vi "Test Method Result String when no Description Provided.vi"(8 "error in (no error)":errorcluster, 11 "Pass Assertion Test In":refnum<class "Method Result Test.lvclass">) -> (0 "error out":errorcluster, 3 "Pass Assertion Test Out":refnum<class "Method Result Test.lvclass">)   [LabVIEW 2020, in "LUnit Tests.lvlib" / "Method Result Test.lvclass"]
uses:
  Method Result Test.lvclass
  66165e44-9c0b-45c8-83e1-30937f51105d.vi
panel:
  out "Result String":string
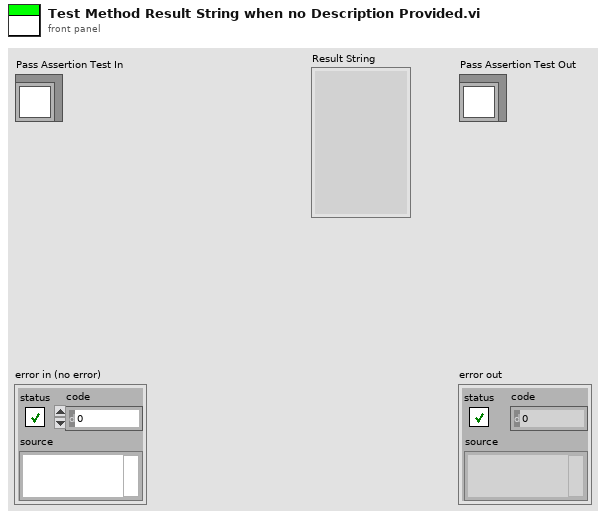
[diagram p1: front panel]
types:
  T1 = typedef "Method Result.lvlib/Method Result.ctl" = cluster{"Test Case":string, "Test Method Name":string, "Status":T2, "Assertion Results":T3[], "Execution time":dbl, "Result String":string}
  T2 = typedef "Assertion Result.lvlib/Status.ctl" = enum16{"Pass", "Fail", "Error", "Skipped", "Setup Error", "Broken", "Teardown Error"}
  T3 = typedef "Assertion Result.lvlib/Assertion Result.ctl" = cluster{"Status":T2, "Message":string, "Description":string, "Assertion Type":T4}
  T4 = typedef "Assertion Result.lvlib/Assertion Type.ctl" = enum16{"None", "Pass", "Fail", "Skip", "Pass if Equal", "Fail if Equal", "Pass if Error", "Fail if Error", "Pass if", "Fail if"}
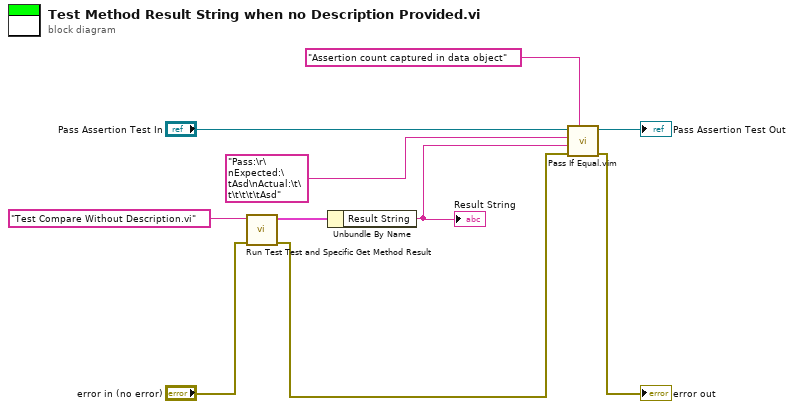
[diagram p0: block diagram]
diagram:
  n1 = call "Run Test Test and Specific Get Method Result.vi"("error in (no error)"="error in (no error)", "Method of Interest"="Test Compare Without Description.vi") -> ("error out"=w3:errorcluster, "Method Result out"=w5:T1)  [unwired: 8 in]
  n2 = Unbundle By Name(w5) -> ("Result String"=w2:string)
  "Result String" <- w2
  n3 = call "Pass If Equal.vim"("Description"="Assertion count captured in data object", "error in (no error)"=w3, "Actual"=w2, "Expected"="Pass:\r\nExpected:\tAsd\nActual:\t\t\t\t\t\tAsd", "LUnit Test Case In"="Pass Assertion Test In") -> ("error out"=→"error out":errorcluster, "LUnit Test Case Out"=→"Pass Assertion Test Out":refnum<class "Method Result Test.lvclass">)  [unwired: 5 in]
